vi "prepare_elec_sensor.vi"(9 "打开":bool=TRUE, 10 "传感器数目":i32=1, 11 "VISA资源名称":refnum<visa-resource-name>) -> ()   [LabVIEW 2017]
uses:
  <vilib>/Instr/_visa.llb/VISA Configure Serial Port (Instr).vi
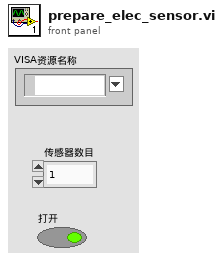
[diagram p1: front panel]
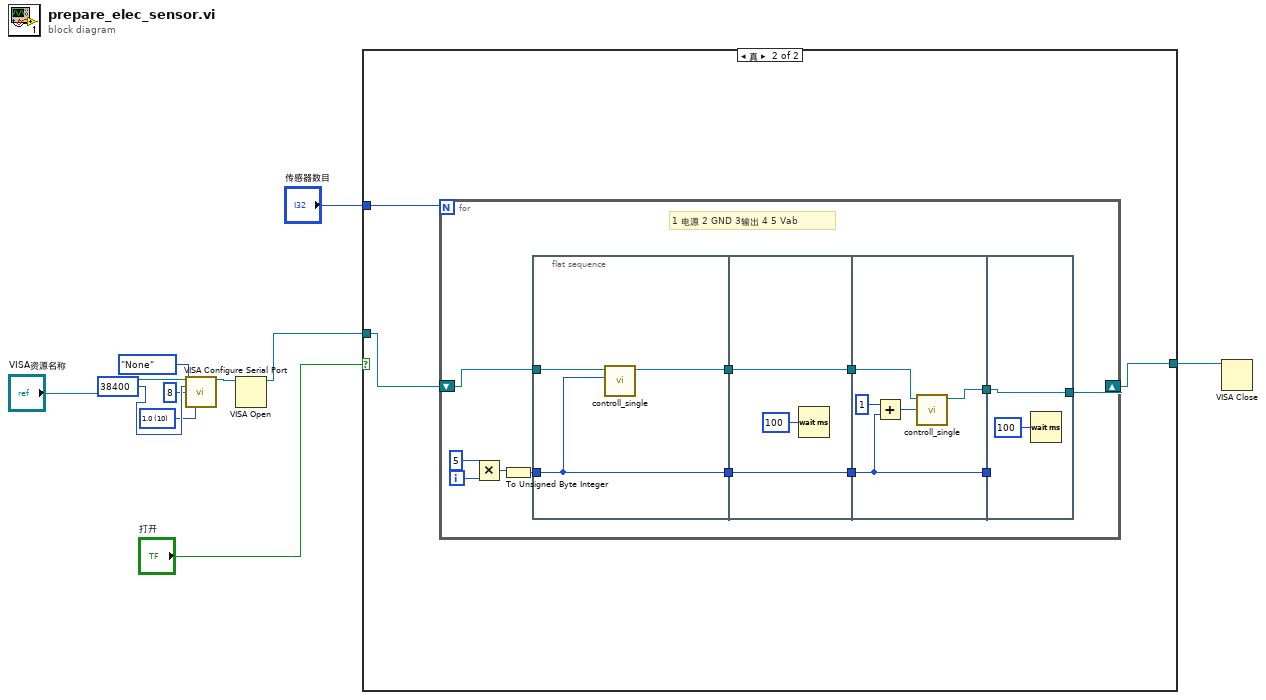
[diagram p0: block diagram]
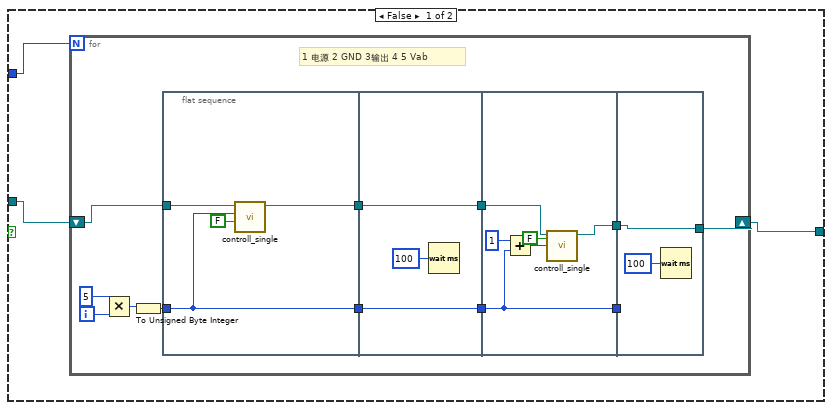
[diagram p2: hidden frame]
diagram:
  w6 = u16 10 items=["1.0"=10, "1.5"=15, "2.0"=20] ("stop bits (10: 1 bit)")
  n1 = call-poly "VISA Configure Serial Port"("VISA resource name"="VISA资源名称", "baud rate (9600)"=u32 38400, "data bits (8)"=u16 8, "parity (0:none)"=enum16{"None", "Odd", "Even", "Mark", "Space"}."None", "stop bits (10: 1 bit)"=w6) -> ("VISA resource name out"=w10:refnum<visa-resource-name>)  [unwired: 9 in, 1 out]
  n2 = VISA Open(VISA resource name=w10) -> (VISA resource name=w5:refnum<visa-resource-name>)  [unwired: 4 in, 1 out]
  n3 = case shown="真" "打开" {
    tunnel: w5 -> [w13 w42]
    tunnel: "传感器数目" -> [w11 w43]
    tunnel: [w12 w41] -> w1
    frame False {
      n4 = for {
        N: w11 -> [_]
        shift-right: [w14] -> w12
        shift-left: w13 -> [w21]
        i -> [w25]
        # "1 电源 2 GND 3输出 4 5 Vab"
        n5 = Multiply(x=5, y=w25) -> (x*y=w23:i32)
        n6 = To Unsigned Byte Integer(number=w23) -> (unsigned 8bit integer=w22:u8)
        n7 = flat-sequence {
          tunnel: w21 -> [w29]
          tunnel: [w28] -> w20
          tunnel: w22 -> [w27]
          tunnel: [w27] -> w18
          tunnel: w20 -> [w32]
          tunnel: [w32] -> w19
          tunnel: w18 -> [w31]
          tunnel: [w31] -> w17
          tunnel: w19 -> [w35]
          tunnel: w17 -> [w37]
          tunnel: [w37] -> w16
          tunnel: [w34] -> w15
          tunnel: w16 -> [_]
          tunnel: w15 -> [w39]
          tunnel: [w39] -> w14
          frame #0 {
            n8 = call "controll_single.vi"("开关"=FALSE, "控制编号"=w27, "VISA资源名称"=w29) -> ("VISA资源名称输出"=w28:refnum<visa-resource-name>)  [unwired: 8 in]
          }
          frame #1 {
            n9 = Wait (ms)(milliseconds to wait=u32 100 ("等待时间（毫秒）")) -> ()  [unwired: 1 out]
          }
          frame #2 {
            n10 = Add(x=u8 1, y=w37) -> (x+y=w36:u8)
            n11 = call "controll_single.vi"("开关"=FALSE, "控制编号"=w36, "VISA资源名称"=w35) -> ("VISA资源名称输出"=w34:refnum<visa-resource-name>)  [unwired: 8 in]
          }
          frame #3 {
            n12 = Wait (ms)(milliseconds to wait=u32 100 ("等待时间（毫秒）")) -> ()  [unwired: 1 out]
          }
        }
      }
    }
    frame True {
      n13 = for {
        N: w43 -> [_]
        shift-right: [w44] -> w41
        shift-left: w42 -> [w51]
        i -> [w55]
        # "1 电源 2 GND 3输出 4 5 Vab"
        n14 = Multiply(x=5, y=w55) -> (x*y=w53:i32)
        n15 = To Unsigned Byte Integer(number=w53) -> (unsigned 8bit integer=w52:u8)
        n16 = flat-sequence {
          tunnel: w51 -> [w58]
          tunnel: [w57] -> w50
          tunnel: w52 -> [w56]
          tunnel: [w56] -> w48
          tunnel: w50 -> [w61]
          tunnel: [w61] -> w49
          tunnel: w48 -> [w60]
          tunnel: [w60] -> w47
          tunnel: w49 -> [w63]
          tunnel: w47 -> [w65]
          tunnel: [w65] -> w46
          tunnel: [w62] -> w45
          tunnel: w46 -> [_]
          tunnel: w45 -> [w67]
          tunnel: [w67] -> w44
          frame #0 {
            n17 = call "controll_single.vi"("控制编号"=w56, "VISA资源名称"=w58) -> ("VISA资源名称输出"=w57:refnum<visa-resource-name>)  [unwired: 9 in]
          }
          frame #1 {
            n18 = Wait (ms)(milliseconds to wait=u32 100 ("等待时间（毫秒）")) -> ()  [unwired: 1 out]
          }
          frame #2 {
            n19 = Add(x=u8 1, y=w65) -> (x+y=w64:u8)
            n20 = call "controll_single.vi"("控制编号"=w64, "VISA资源名称"=w63) -> ("VISA资源名称输出"=w62:refnum<visa-resource-name>)  [unwired: 9 in]
          }
          frame #3 {
            n21 = Wait (ms)(milliseconds to wait=u32 100 ("等待时间（毫秒）")) -> ()  [unwired: 1 out]
          }
        }
      }
    }
  }
  n22 = VISA Close(VISA resource name=w1) -> ()  [unwired: 1 in, 1 out]
